vi "New.vi"(8 "error in (no error)":errorcluster, 11 "reference in":refnum<class "suite SSL Client.lvclass">) -> (0 "error out":errorcluster, 3 "reference out":refnum<class "suite SSL Client.lvclass">)   [LabVIEW 2013, in "suite SSL Client.lvclass"]
uses:
  suite SSL Client.lvclass
  <vilib>/addons/_JKI Toolkits/VI Tester/TestSuite.llb/TestSuite.lvclass
  <vilib>/addons/_JKI Toolkits/VI Tester/TestCase.llb/TestCase.lvclass
  test SSL Client/test SSL Client.lvclass
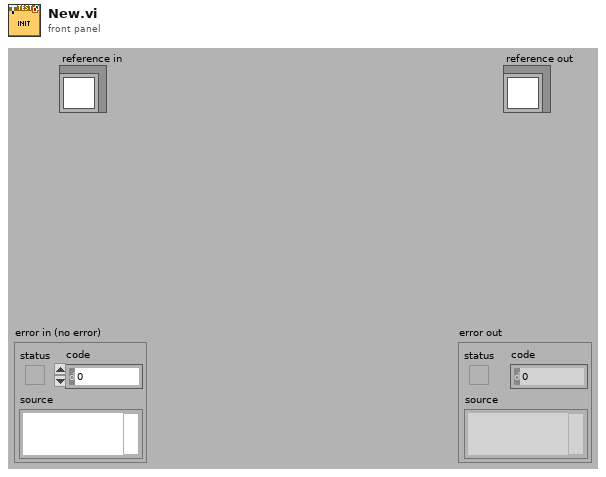
[diagram p1: front panel]
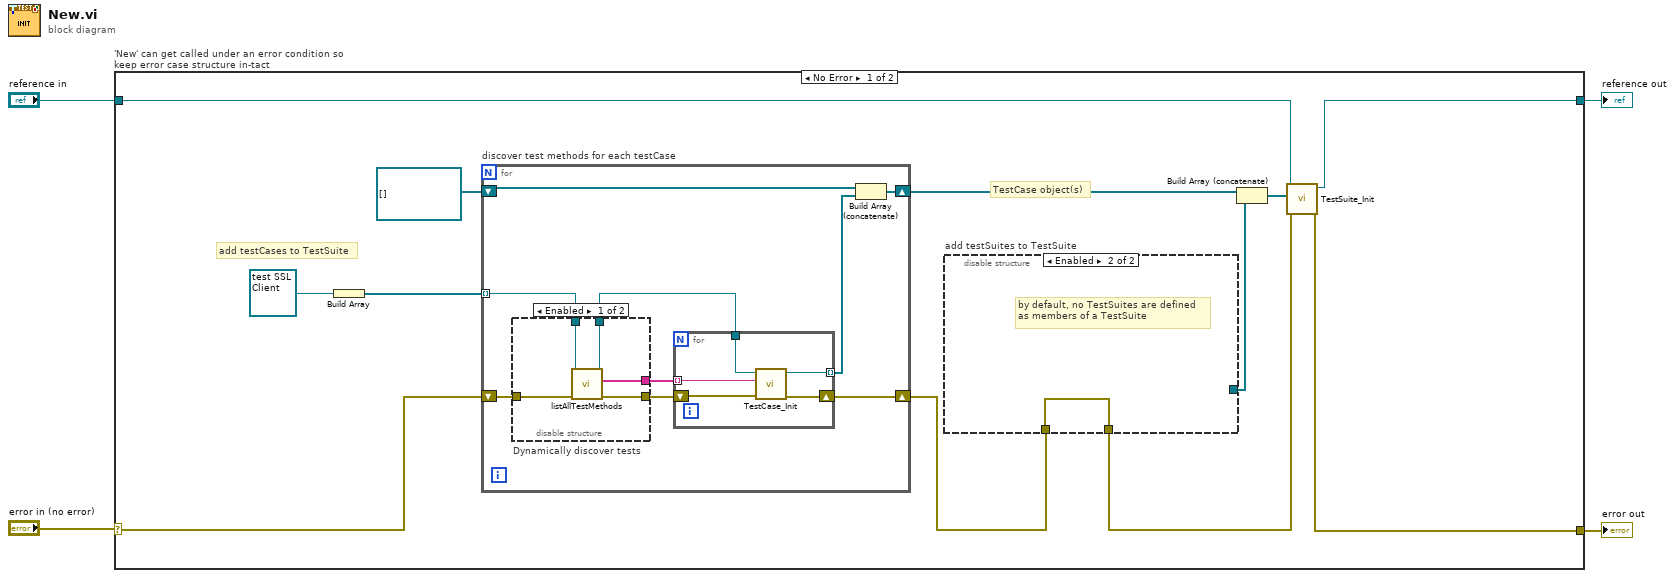
[diagram p0: block diagram]
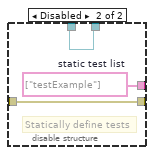
[diagram p2: hidden frame]
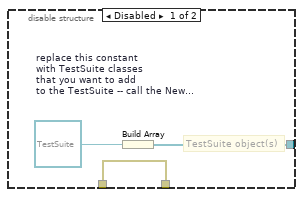
[diagram p3: hidden frame]
diagram:
  n1 = case "'New' can get called under an error condition so keep error case structure in-tact" shown="No Error" "error in (no error)" {
    selector: "error in (no error)" -> [w12 w43]
    tunnel: [w16 w44] -> w4
    tunnel: "reference in" -> [w13 w44]
    tunnel: [w15 w43] -> w1
    frame No Error {
      # "TestCase object(s)"
      # "add testCases to TestSuite"
      n2 = Build Array(refnum<class "test SSL Client.lvclass"> refnum ("test SSL Client.lvclass")) -> (w14:refnum<class "test SSL Client.lvclass">[])
      n3 = for "discover test methods for each testCase" {
        shift-right: [w25] -> w7
        shift-left: w12 -> [w21]
        tunnel: w14 -> [w18] mode=indexing
        shift-right: [w22] -> w11
        shift-left: refnum<class "TestCase.lvclass">[] [] -> [w23]
        n4 = disable-structure "Dynamically discover tests" shown="Enabled" {
          disable-tunnel: w21 -> [w30 w31]
          disable-tunnel: [w29 w31] -> w20
          disable-tunnel: [w28 w32] -> w19
          disable-tunnel: w18 -> [w27 w33]
          disable-tunnel: [w26 w33] -> w17
          frame Enabled {
            n5 = call-dynamic "listAllTestMethods.vi"("error in (no error)"=w30, "TestCase in"=w27) -> ("error out"=w29:errorcluster, "test methods"=w28:string[], "TestCase out"=w26:refnum<class "test SSL Client.lvclass">)  [unwired: 7 in]
          }
          frame Disabled {
            w32 = string[] ["testExample"]  # static test list
            # "Statically define tests"
          }
        }
        n6 = for {
          tunnel: w17 -> [w34]
          tunnel: w19 -> [w38] mode=indexing
          shift-right: [w36] -> w25
          shift-left: w20 -> [w37]
          tunnel: [w35] -> w24 mode=indexing
          n7 = call <vilib>:"TestCase_Init.vi"("error in (no error)"=w37, "methodName (\"runTest\")"=w38, "TestCase in"=w34) -> ("error out"=w36:errorcluster, "TestCase out"=w35:refnum<class "test SSL Client.lvclass">)  [unwired: 7 in]
        }
        n8 = Build Array (concatenate)(w23, w24) -> (w22:refnum<class "TestCase.lvclass">[])
      }
      n9 = disable-structure "add testSuites to TestSuite" shown="Enabled" {
        disable-tunnel: [w39 _] -> w9
        disable-tunnel: [w41 w42] -> w8
        disable-tunnel: w7 -> [w41 w42]
        frame Disabled {
          w40 = refnum<class "TestSuite.lvclass"> refnum  # replace this constant with TestSuite classes that you want to add to the TestSuite -- call the New method for each TestSuite prior to adding it to this TestSuite
          # "TestSuite object(s)"
          n10 = Build Array(w40) -> (w39:refnum<class "TestSuite.lvclass">[])
        }
        frame Enabled {
          # "by default, no TestSuites are defined\nas members of a TestSuite"
        }
      }
      n11 = Build Array (concatenate)(w11, w9) -> (w10:refnum<class>[])
      n12 = call <vilib>:"TestSuite_Init.vi"("error in (no error)"=w8, "tests (none)"=w10, "TestSuite in"=w13) -> ("error out"=w15:errorcluster, "TestSuite out"=w16:refnum<class "suite SSL Client.lvclass">)  [unwired: 7 in]
    }
    frame Error {
    }
  }
  "reference out" <- w4
  "error out" <- w1
